vi "Single SSC DCPower Configure Settings.vi"(0 "DCPower SSC in":T3, 1 "Aperture Time Units (Seconds)":T2=1028 items=["Seconds"=1028, "Powerline Cycles"=1029], 2 "Transient Response (Normal)":i32(ring)=1038 items=["Slow"=1041, "Normal"=1038, "Fast"=1039, "Custom"=1042], 5 "Aperture Time (16.6m)":dbl=0.01666666666 format="%#_6p", 7 "Source Delay (0 seconds)":dbl format="%#_6p", 9 "Sense (Local)":T1=1008 items=["Local"=1008, "Remote"=1009], 11 "error in":errorcluster) -> (4 "DCPower SSC out":T3, 15 "error out":errorcluster)   [LabVIEW 2019]
doc: "This VI configures important DCPower channel settings for a session.\n\nSettings are ignored if they aren't supported by the device being used."
uses:
  SSC DCPower.ctl
  <instrlib>/niDCPower/nidcpower.llb/niDCPower Aperture Time Units.ctl
  <instrlib>/niDCPower/nidcpower.llb/niDCPower Sense.ctl
  SSC DCPower Debug Global.vi
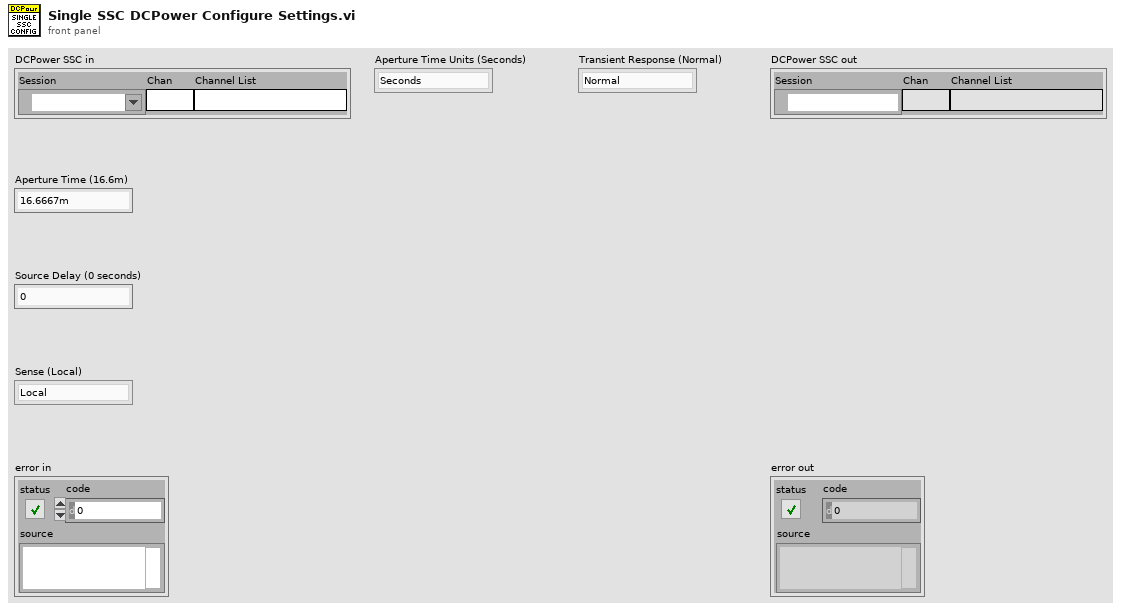
[diagram p1: front panel]
types:
  T1 = typedef "niDCPower Sense.ctl" = i32
  T2 = typedef "niDCPower Aperture Time Units.ctl" = i32
  T3 = typedef "SSC DCPower.ctl" = cluster{"Session":refnum<k15>, "Chan":string, "Channel List":string}
  T4 = typedef "niDCPower Power Line Frequency.ctl" = dbl
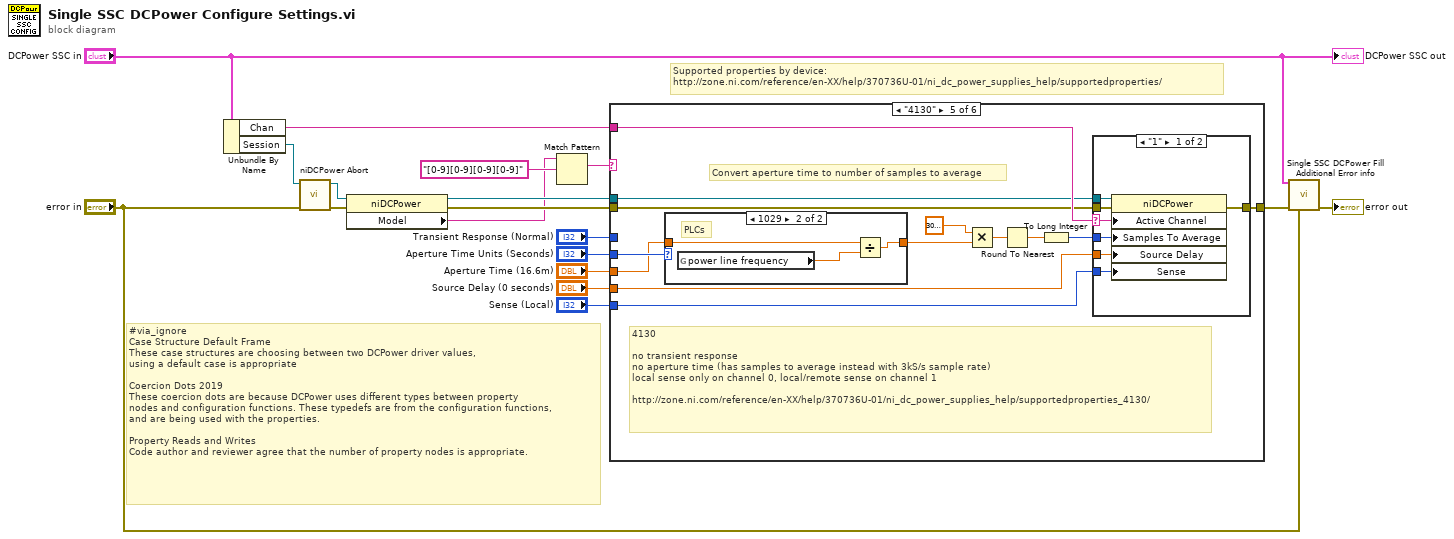
[diagram p0: block diagram]
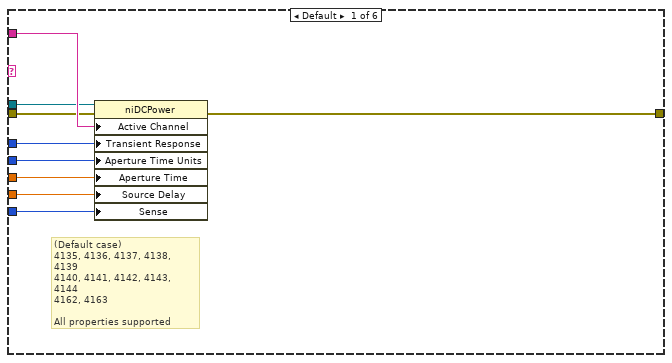
[diagram p2: hidden frame]
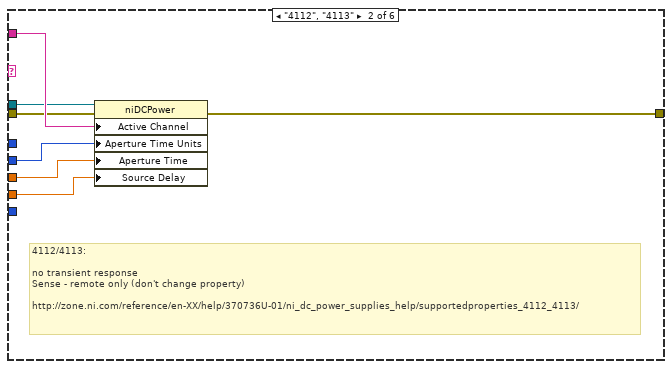
[diagram p3: hidden frame]
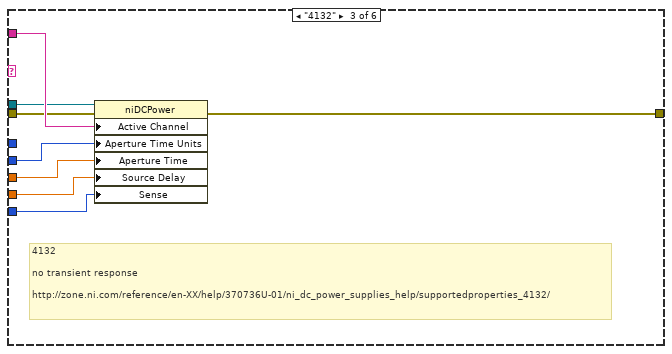
[diagram p4: hidden frame]
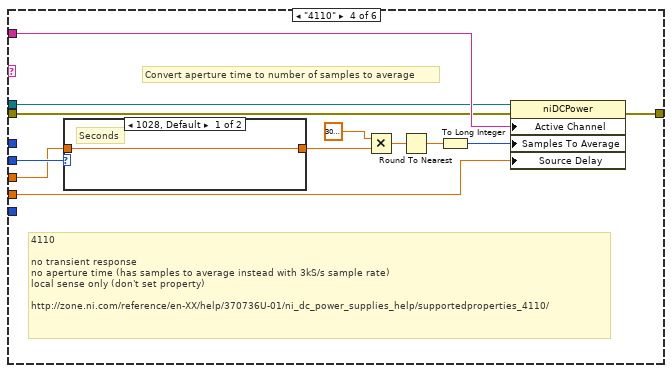
[diagram p5: hidden frame]
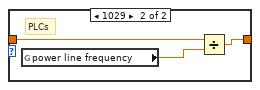
[diagram p6: hidden frame]
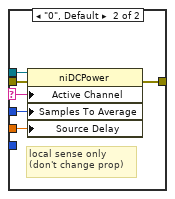
[diagram p7: hidden frame]
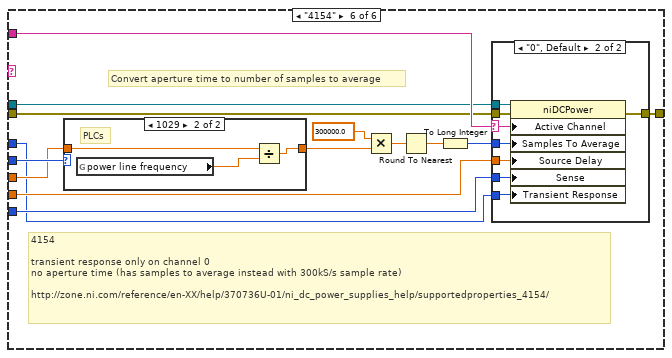
[diagram p9: hidden frame]
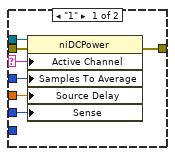
[diagram p10: hidden frame]
diagram:
  # "#via_ignore \nCase Structure Default Frame\nThese case structures are choosing between two DCPower driver values,\nusing a default case is appropriate\n\nCoercion Dots 2019\nThese coercion dots are because DCPower uses different types between property\nnodes and configuration functions. These typedefs are from the configuration functions, \nand are being used with the properties.\n\nProperty Reads and Writes\nCode author and reviewer agree that the number of property nodes is appropriate."
  # "Supported properties by device:\nhttp://zone.ni.com/reference/en-XX/help/370736U-01/ni_dc_power_supplies_help/supportedproperties/"
  n1 = Unbundle By Name("DCPower SSC in") -> ("Chan"=w17:string, "Session"=w7:refnum<k15>)
  n2 = call <instrlib>:"niDCPower Abort.vi"("error in (no error)"="error in", "instrument handle"=w7) -> ("error out"=w11:errorcluster, "instrument handle out"=w9:refnum<k15>)  [unwired: 8 in]
  n3 = property class="niDCPower"(reference=w9, error in=w11) -> (reference out=w8:refnum<k15>, error out=w10:errorcluster, "Model"=w5:string)
  n4 = Match Pattern(string=w5, regular expression="[0-9][0-9][0-9][0-9]") -> (match substring=w4:string)  [unwired: 1 in, 3 out]
  n5 = case shown="\"4130\"" w4 {
    tunnel: [w27 w34 w42 w54 w71 w102] -> w18
    tunnel: w17 -> [w26 w33 w41 w53 w70 w101]
    tunnel: "Transient Response (Normal)" -> [w25 _ _ _ _ w89]
    tunnel: "Aperture Time Units (Seconds)" -> [w24 w32 w40 w49 w65 w96]
    tunnel: "Aperture Time (16.6m)" -> [w23 w31 w39 w48 w64 w95]
    tunnel: "Source Delay (0 seconds)" -> [w22 w30 w38 w52 w69 w100]
    tunnel: "Sense (Local)" -> [w21 _ w35 _ w68 w99]
    tunnel: w10 -> [w20 w29 w37 w51 w67 w98]
    tunnel: w8 -> [w19 w28 w36 w50 w66 w97]
    frame Default {
      # "(Default case)\n4135, 4136, 4137, 4138, 4139\n4140, 4141, 4142, 4143, 4144\n4162, 4163\n\nAll properties supported"
      n6 = property class="niDCPower"(reference=w19, error in=w20, "Active Channel"=w26, "Transient Response"=w25, "Aperture Time Units"=w24, "Aperture Time"=w23, "Source Delay"=w22, "Sense"=w21) -> (error out=w27:errorcluster)  [unwired: 1 out]
    }
    frame "4112", "4113" {
      # "4112/4113:\n\nno transient response\nSense - remote only (don't change property)\n\nhttp://zone.ni.com/reference/en-XX/help/370736U-01/ni_dc_power_supplies_help/supportedproperties_4112_4113/"
      n7 = property class="niDCPower"(reference=w28, error in=w29, "Active Channel"=w33, "Aperture Time Units"=w32, "Aperture Time"=w31, "Source Delay"=w30) -> (error out=w34:errorcluster)  [unwired: 1 out]
    }
    frame "4132" {
      # "4132\n\nno transient response\n\nhttp://zone.ni.com/reference/en-XX/help/370736U-01/ni_dc_power_supplies_help/supportedproperties_4132/"
      n8 = property class="niDCPower"(reference=w36, error in=w37, "Active Channel"=w41, "Aperture Time Units"=w40, "Aperture Time"=w39, "Source Delay"=w38, "Sense"=w35) -> (error out=w42:errorcluster)  [unwired: 1 out]
    }
    frame "4110" {
      # "Convert aperture time to number of samples to average"
      # "4110\n\nno transient response\nno aperture time (has samples to average instead with 3kS/s sample rate)\nlocal sense only (don't set property)\n\nhttp://zone.ni.com/reference/en-XX/help/370736U-01/ni_dc_power_supplies_help/supportedproperties_4110/"
      n9 = case shown="1028, Default" w49 {
        tunnel: w48 -> [w55 w58]
        tunnel: [w55 w56] -> w47
        frame 1028, Default {
          # "Seconds"
        }
        frame 1029 {
          # "PLCs"
          n10 = global read "SSC DCPower Debug Global.vi" "power line frequency"() -> (w57:T4)
          n11 = Divide(x=w58, y=w57) -> (x/y=w56:T4)
        }
      }
      n12 = Multiply(x=3000.0, y=w47) -> (x*y=w46:T4)
      n13 = Round To Nearest(number=w46) -> (nearest integer value=w45:T4)
      n14 = To Long Integer(number=w45) -> (32bit integer=w43:i32)
      n15 = property class="niDCPower"(reference=w50, error in=w51, "Active Channel"=w53, "Samples To Average"=w43, "Source Delay"=w52) -> (error out=w54:errorcluster)  [unwired: 1 out]
    }
    frame "4130" {
      # "Convert aperture time to number of samples to average"
      # "4130\n\nno transient response\nno aperture time (has samples to average instead with 3kS/s sample rate)\nlocal sense only on channel 0, local/remote sense on channel 1\n\nhttp://zone.ni.com/reference/en-XX/help/370736U-01/ni_dc_power_supplies_help/supportedproperties_4130/"
      n16 = case shown="1029" w65 {
        tunnel: w64 -> [w85 w88]
        tunnel: [w85 w86] -> w63
        frame 1028, Default {
          # "Seconds"
        }
        frame 1029 {
          # "PLCs"
          n17 = global read "SSC DCPower Debug Global.vi" "power line frequency"() -> (w87:T4)
          n18 = Divide(x=w88, y=w87) -> (x/y=w86:T4)
        }
      }
      n19 = Multiply(x=3000.0, y=w63) -> (x*y=w62:T4)
      n20 = Round To Nearest(number=w62) -> (nearest integer value=w61:T4)
      n21 = To Long Integer(number=w61) -> (32bit integer=w59:i32)
      n22 = case shown="\"1\"" w70 {
        selector: w70 -> [w77 w83]
        tunnel: [w78 w84] -> w71
        tunnel: w69 -> [w76 w82]
        tunnel: w68 -> [w75 _]
        tunnel: w67 -> [w74 w81]
        tunnel: w66 -> [w73 w80]
        tunnel: w59 -> [w72 w79]
        frame "1" {
          n23 = property class="niDCPower"(reference=w73, error in=w74, "Active Channel"=w77, "Samples To Average"=w72, "Source Delay"=w76, "Sense"=w75) -> (error out=w78:errorcluster)  [unwired: 1 out]
        }
        frame "0", Default {
          # "local sense only\n(don't change prop)"
          n24 = property class="niDCPower"(reference=w80, error in=w81, "Active Channel"=w83, "Samples To Average"=w79, "Source Delay"=w82) -> (error out=w84:errorcluster)  [unwired: 1 out]
        }
      }
    }
    frame "4154" {
      # "4154\n\ntransient response only on channel 0\nno aperture time (has samples to average instead with 300kS/s sample rate)\n\nhttp://zone.ni.com/reference/en-XX/help/370736U-01/ni_dc_power_supplies_help/supportedproperties_4154/"
      # "Convert aperture time to number of samples to average"
      n25 = case shown="1029" w96 {
        tunnel: w95 -> [w118 w121]
        tunnel: [w118 w119] -> w94
        frame 1028, Default {
          # "Seconds"
        }
        frame 1029 {
          # "PLCs"
          n26 = global read "SSC DCPower Debug Global.vi" "power line frequency"() -> (w120:T4)
          n27 = Divide(x=w121, y=w120) -> (x/y=w119:T4)
        }
      }
      n28 = Multiply(x=300000.0, y=w94) -> (x*y=w93:T4)
      n29 = Round To Nearest(number=w93) -> (nearest integer value=w92:T4)
      n30 = To Long Integer(number=w92) -> (32bit integer=w90:i32)
      n31 = case shown="\"0\", Default" w101 {
        selector: w101 -> [w108 w116]
        tunnel: [w109 w117] -> w102
        tunnel: w100 -> [w107 w115]
        tunnel: w99 -> [w106 w111]
        tunnel: w98 -> [w105 w114]
        tunnel: w97 -> [w104 w113]
        tunnel: w90 -> [w103 w112]
        tunnel: w89 -> [_ w110]
        frame "1" {
          n32 = property class="niDCPower"(reference=w104, error in=w105, "Active Channel"=w108, "Samples To Average"=w103, "Source Delay"=w107, "Sense"=w106) -> (error out=w109:errorcluster)  [unwired: 1 out]
        }
        frame "0", Default {
          n33 = property class="niDCPower"(reference=w113, error in=w114, "Active Channel"=w116, "Samples To Average"=w112, "Source Delay"=w115, "Sense"=w111, "Transient Response"=w110) -> (error out=w117:errorcluster)  [unwired: 1 out]
        }
      }
    }
  }
  n34 = call "Single SSC DCPower Fill Additional Error info.vi"("DCPower SSC in"="DCPower SSC in", "error in"=w18, "previous error in"="error in") -> ("error out"=→"error out":errorcluster)  [unwired: 12 in]
  "DCPower SSC out" <- "DCPower SSC in"
